vi "Initialize.vi"(8 "error in (no error)":errorcluster) -> (0 "error out":errorcluster)   [LabVIEW 2009, in "HighFinesse WS5.lvlib"]
doc: "Starts the wavelength meter program in hidden mode (if it's not already running) and sets some default measurement values. To ensure a consistent state for later VIs, call this VI before calling other instrument driver VIs for this instrument. Generally, you need to call the Initialize VI only once at the beginning of an application."
uses:
  HighFinesse WS5.lvlib
  Variable Typedefs.llb/Exposure Mode.ctl
  Control typedefs.llb/Control Action.ctl
  Configure/Operation.vi
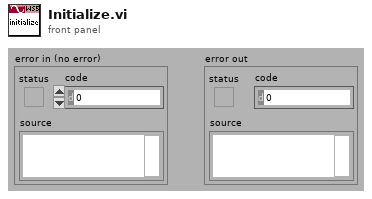
[diagram p1: front panel]
types:
  T1 = typedef "Control Action.ctl" = u32
  T2 = typedef "HighFinesse WS5.lvlib/Exposure Mode.ctl" = enum16{"manual", "automatic"}
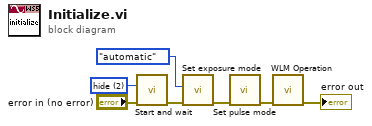
[diagram p0: block diagram]
diagram:
  w1 = T1 2 items=["show"=1, "hide"=2, "exit"=3] ("command (show)")
  n1 = call "Start and wait.vi"("error in (no error)"="error in (no error)", "command (show)"=w1) -> ("error out"=w7:errorcluster)  [unwired: 9 out]
  n2 = call "Set exposure mode.vi"("error in (no error)"=w7, "exposure mode"=Exposure_Mode."automatic") -> ("error out"=w5:errorcluster)  [unwired: 9 out]
  n3 = call "Set pulse mode.vi"("error in (no error)"=w5) -> ("error out"=w4:errorcluster)  [unwired: 1 in, 9 out]
  n4 = call "WLM Operation.vi"("error in (no error)"=w4) -> ("error out"=→"error out":errorcluster)  [unwired: 1 in, 9 out]
